vi "Init Data.vi"(8 "error in (no error)":errorcluster, 10 "Data Object":refnum<class "Factory Plugin Framework.lvclass">=refnum, 11 "File Parser Interface in":refnum<class "File Parser Interface.lvclass">) -> (0 "error out":errorcluster, 3 "File Parser Interface out":refnum<class "File Parser Interface.lvclass">)   [LabVIEW 2018, in "File Parser Interface.lvlib" / "File Parser Interface.lvclass"]
uses:
  File Parser Interface.lvclass
  FPF.lvlibp/Factory Plugin Framework.lvclass
  File Parser Interface.lvclass/File Parser Interface.ctl
  Read File Path.vi
  Read Protocol Type.vi
  Write File Path.vi
  Write Protocol Type.vi
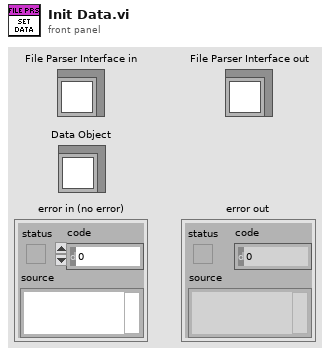
[diagram p1: front panel]
types:
  T1 = typedef "Protocol Type.ctl" = enum16{"BML_LS", "BML_HS", "SPI_3W", "SPI_4W"}
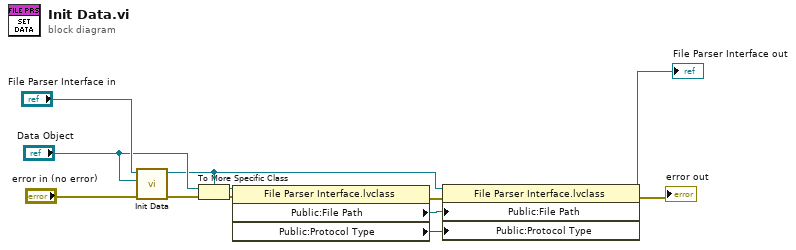
[diagram p0: block diagram]
diagram:
  n1 = call-parent "Init Data.vi"("error in (no error)"="error in (no error)", "Data Object"="Data Object", "Factory Plugin Framework in"="File Parser Interface in") -> ("error out"=w10:errorcluster, "Factory Plugin Framework out"=w6:refnum<class "File Parser Interface.lvclass">)  [unwired: 7 in]
  n2 = To More Specific Class(target class=w6, reference="Data Object", error in=w10) -> (specific class reference=w7:refnum<class "File Parser Interface.lvclass">, error out=w8:errorcluster)
  n3 = property class="File Parser Interface.lvclass"(reference=w7, error in=w8) -> (error out=w5:errorcluster, "Public:File Path"=w4:path, "Public:Protocol Type"=w1:T1)  [unwired: 1 out]
  n4 = property class="File Parser Interface.lvclass"(reference=w6, error in=w5, "Public:File Path"=w4, "Public:Protocol Type"=w1) -> (reference out=→"File Parser Interface out":refnum<class "File Parser Interface.lvclass">, error out=→"error out":errorcluster)
